vi "UDP Discovery Server (subnet).vi"(0 "Name":string, 5 "port":u16=10000, 7 "TCP Port":u16, 9 "send full address":bool) -> (15 "error out":errorcluster)   [LabVIEW 2020]
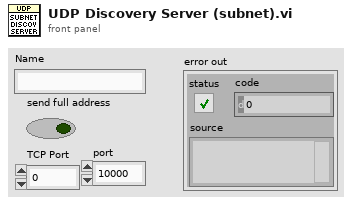
[diagram p1: front panel]
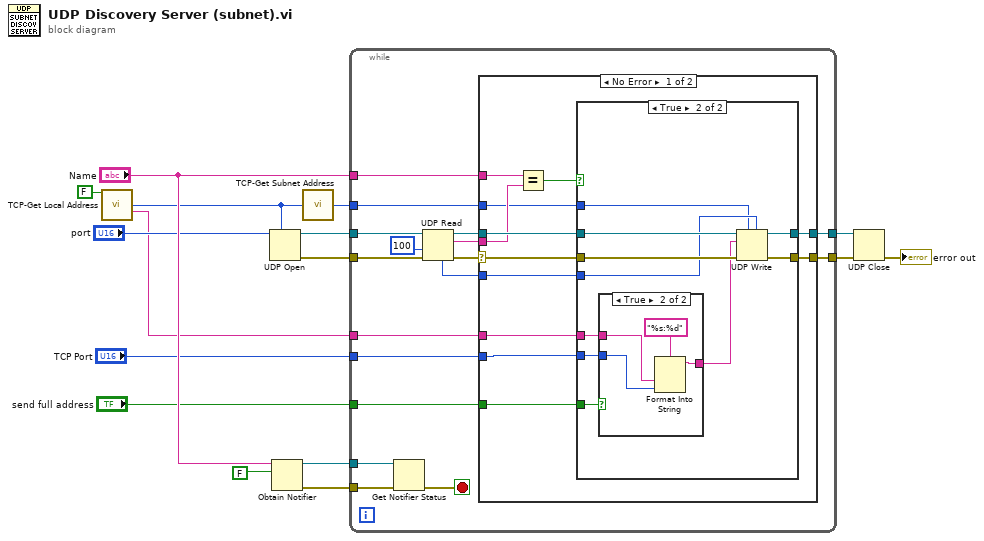
[diagram p0: block diagram]
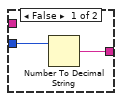
[diagram p3: hidden frame]
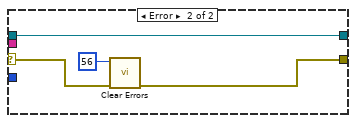
[diagram p4: hidden frame]
diagram:
  n1 = call "TCP-Get Local Address.vi"("LAN first"=FALSE) -> ("net address"=w5:u32, "address"=w2:string)  [unwired: 13 in]
  n2 = UDP Open(7:w5, 11:"port") -> (port=w13:refnum<k16>, 0:w14:errorcluster)  [unwired: 3 in, 1 out]
  n3 = Obtain Notifier(name (unnamed)="Name", notification data type=FALSE) -> (notifier out=w9:refnum<notifier>, error out=w8:errorcluster)  [unwired: 2 in, 1 out]
  n4 = call "TCP-Get Subnet Address.vi"("net address"=w5) -> ("subnet address"=w4:u32)  [unwired: 13 in, 1 out]
  n5 = while {
    tunnel: w13 -> [w33]
    tunnel: w14 -> [w32]
    tunnel: [w31] -> w15
    tunnel: [w30] -> w16
    tunnel: "Name" -> [w29]
    tunnel: "TCP Port" -> [w23]
    tunnel: w9 -> [w22]
    tunnel: w8 -> [w21]
    tunnel: w4 -> [w19]
    tunnel: w2 -> [w18]
    tunnel: "send full address" -> [w17]
    stop <- w20 stop-if-true
    n6 = Get Notifier Status(notifier=w22, error in (no error)=w21) -> (error out=w20:errorcluster)  [unwired: 4 out]
    n7 = UDP Read(connection ID=w33, timeout ms (25000)=100, 8:w32) -> (data out=w26:string, error out=w27:errorcluster, 3:w25:refnum<k16>, 4:w24:u16)  [unwired: 2 out]
    n8 = case shown="No Error" w27 {
      selector: w27 -> [w41 w67]
      tunnel: [w42 w65] -> w31
      tunnel: w26 -> [w40 _]
      tunnel: w29 -> [w45 _]
      tunnel: w25 -> [w44 w64]
      tunnel: [w43 w64] -> w30
      tunnel: w24 -> [w39 _]
      tunnel: w23 -> [w34 _]
      tunnel: w19 -> [w37 _]
      tunnel: w18 -> [w36 _]
      tunnel: w17 -> [w35 _]
      frame No Error {
        n9 = Equal?(x=w45, y=w40) -> (x = y?=w38:bool)
        n10 = case shown="True" w38 {
          tunnel: w44 -> [w47 w57]
          tunnel: [w47 w56] -> w43
          tunnel: [w46 w55] -> w42
          tunnel: w41 -> [w46 w54]
          tunnel: w39 -> [_ w53]
          tunnel: w37 -> [_ w52]
          tunnel: w36 -> [_ w48]
          tunnel: w35 -> [_ w51]
          tunnel: w34 -> [_ w50]
          frame False {
          }
          frame True {
            n11 = case shown="True" w51 {
              tunnel: w50 -> [w59 w61]
              tunnel: [w58 w63] -> w49
              tunnel: w48 -> [_ w62]
              frame False {
                n12 = Number To Decimal String(number=w59) -> (decimal integer string=w58:string)  [unwired: 1 in]
              }
              frame True {
                n13 = Format Into String(format string="%s:%d", w62, w61) -> (resulting string=w63:string)  [unwired: 2 in, 1 out]
              }
            }
            n14 = UDP Write(address=w52, port or service name=w53, connection ID=w57, data in=w49, 8:w54) -> (error out=w55:errorcluster, 3:w56:refnum<k16>)  [unwired: 1 in]
          }
        }
      }
      frame Error {
        n15 = call <vilib>:"Clear Errors.vi"("error in (no error)"=w67, "specific error code to clear (0: all)"=56) -> ("error out"=w65:errorcluster)  [unwired: 4 in, 1 out]
      }
    }
  }
  n16 = UDP Close(connection ID=w16, 8:w15) -> (error out=→"error out":errorcluster)  [unwired: 1 out]
